vi "15-ParseInput.vi"(11 "String":string) -> (3 "Risk Array":u8[][](array[numeric]))   [LabVIEW 2019, in "15.lvlib"]
uses:
  15.lvlib
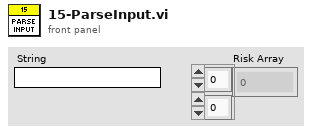
[diagram p1: front panel]
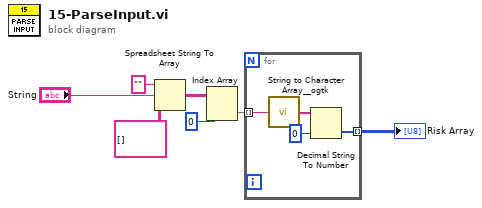
[diagram p0: block diagram]
diagram:
  n1 = Spreadsheet String To Array(format string="", spreadsheet string="String", array type (2D Dbl)=string[][] [] ("format string")) -> (array=w3:string[][])  [unwired: 1 in]
  n2 = Index Array(array=w3, index (col)=0 ("disabled index (col)")) -> (element=w4:string[])  [unwired: 1 in]
  n3 = for {
    tunnel: w4 -> [w11] mode=indexing
    tunnel: [w8] -> w7 mode=indexing
    n4 = call <userlib>:"String to Character Array__ogtk.vi"("Input String"=w11) -> ("Character Array"=w10:string[])
    n5 = Decimal String To Number(string=w10, default (0L)=u8 0 ("default (0 I32)")) -> (number=w8:u8[])  [unwired: 1 in, 1 out]
  }
  "Risk Array" <- w7
